vi "Force wench motor to one direction and stop when limit switch pressed.vi"(10 "Limit switch input":bool, 11 "Wench motor input":dbl) -> (3 "Wench Motor outut":dbl)   [LabVIEW 2013]
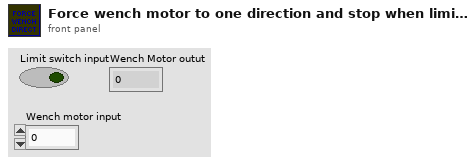
[diagram p1: front panel]
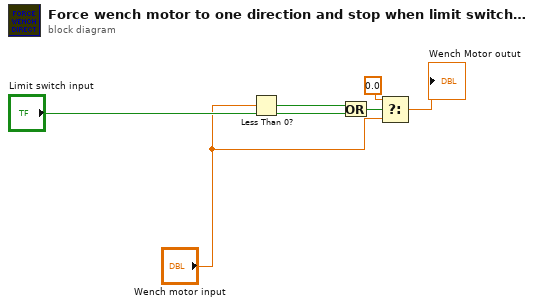
[diagram p0: block diagram]
diagram:
  n1 = Less Than 0?(x="Wench motor input") -> (x < 0?=w6:bool)
  n2 = Or(x=w6, y="Limit switch input") -> (x .or. y?=w4:bool)
  n3 = Select(t=0.0, s=w4, f="Wench motor input") -> (s? t:f=→"Wench Motor outut":dbl)
